vi "DSF.Engine.Plugin.Set Plugin Runtime.vi"(8 "error in (no error)":errorcluster, 10 "Plugin Runtime":refnum<class "DSF.Engine.Runtime.Plugin.lvclass">, 11 "Plugin in":refnum<class "Plugin.lvclass">) -> (0 "error out":errorcluster, 3 "Plugin out":refnum<class "Plugin.lvclass">)   [LabVIEW 2016, in "DSF.Engine.lvlib" / "Plugin.lvclass"]
uses:
  Plugin.lvclass
  DSF.Engine.Runtime.Plugin.lvclass
  Plugin.lvclass/Plugin.ctl
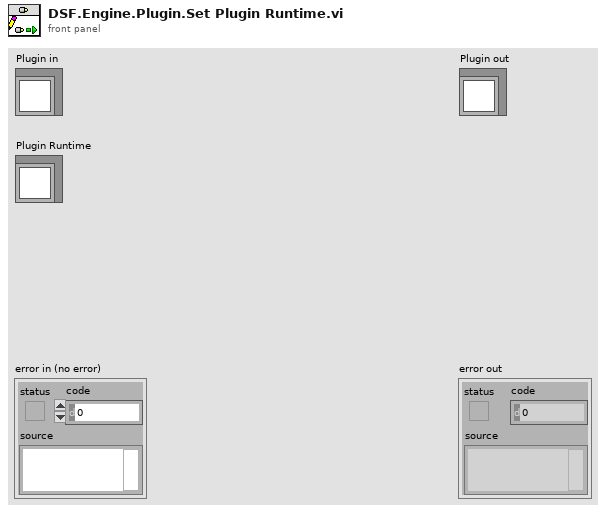
[diagram p1: front panel]
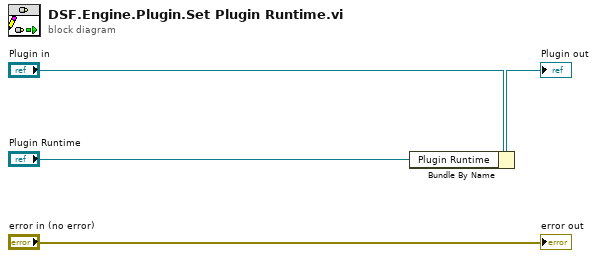
[diagram p0: block diagram]
diagram:
  n1 = Bundle By Name(cluster="Plugin in", "Plugin Runtime"="Plugin Runtime") -> (→"Plugin out":refnum<class "Plugin.lvclass">)
  "error out" <- "error in (no error)"
